vi "ReadIV.vi"(8 "error in (no error)":errorcluster, 9 "Chan":i32, 11 "reference in":refnum<class "PSU_Keysight_34951A.lvclass">) -> (0 "error out":errorcluster, 1 "V":dbl, 2 "I":dbl, 3 "reference in":refnum<class "PSU_Keysight_34951A.lvclass">)   [LabVIEW 2022 SP3, in "PSU_Keysight_34951A.lvlib" / "PSU_Keysight_34951A.lvclass"]
uses:
  PSU_Keysight_34951A.lvclass
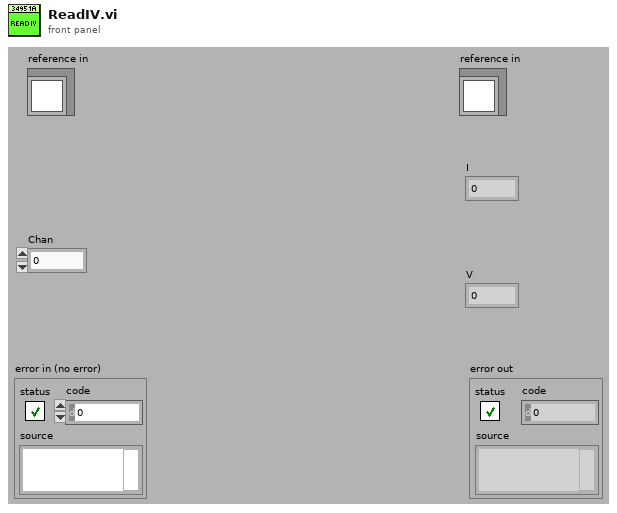
[diagram p1: front panel]
types:
  T1 = typedef "PSU_Keysight_34951A.lvlib/PSU_Keysight_34951A.lvclass/ObjectAttributes.ctl" = cluster{"Config":T2, "VISA res":refnum<visa-resource-name>, "Enabled":bool[], "V":dbl[], "I":dbl[], "Source Type":enum16{"Voltage", "Current"}[]}
  T2 = typedef "PSU_Keysight_34951A.lvlib/PSU_Keysight_34951A.lvclass/Config.ctl" = cluster{"VISA":refnum<visa-resource-name>, "Slot":i32}
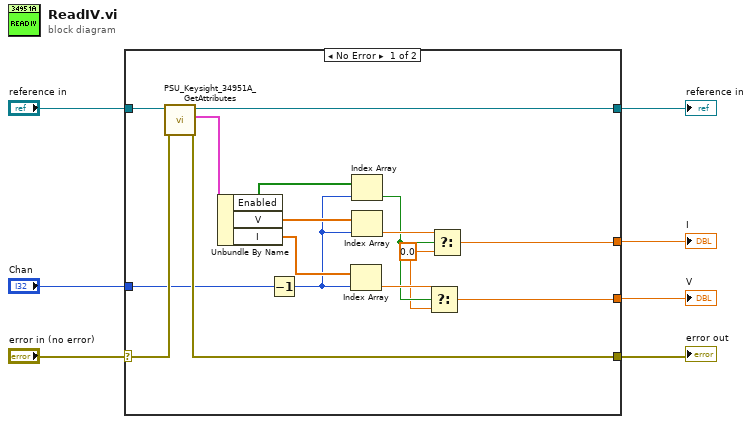
[diagram p0: block diagram]
diagram:
  n1 = case shown="No Error" "error in (no error)" {
    selector: "error in (no error)" -> [w23 w25]
    tunnel: [w21 w25] -> w6
    tunnel: [w19 w24] -> w4
    tunnel: "reference in" -> [w20 w24]
    tunnel: "Chan" -> [w17 _]
    tunnel: [w9 _] -> w2
    tunnel: [w8 _] -> w1
    frame No Error {
      w10 = 0.0 ("f")
      n2 = call "PSU_Keysight_34951A_GetAttributes.vi"("error in (no error)"=w23, "reference in"=w20) -> ("error out"=w21:errorcluster, "Data"=w22:T1, "reference out"=w19:refnum<class "PSU_Keysight_34951A.lvclass">)  [unwired: 6 in, 1 out]
      n3 = Unbundle By Name(w22) -> ("Enabled"=w14:bool[], "V"=w18:dbl[], "I"=w16:dbl[])
      n4 = Decrement(x=w17) -> (x-1=w15:i32)
      n5 = Index Array(array=w16, index=w15) -> (element=w12:dbl)
      n6 = Index Array(array=w14, index=w15) -> (element=w11:bool)
      n7 = Index Array(array=w18, index=w15) -> (element=w13:dbl)
      n8 = Select(t=w12, s=w11, f=w10) -> (s? t:f=w8:dbl)
      n9 = Select(t=w13, s=w11, f=w10) -> (s? t:f=w9:dbl)
    }
    frame Error {
    }
  }
  "error out" <- w6
  "reference in" <- w4
  "I" <- w2
  "V" <- w1
